vi "Warning Edit.vi"(10 "Data Path":path, 11 "Project":string) -> (2 "Warning Data":string[][](array[string]), 3 "OK?":bool)   [LabVIEW 2020]
uses:
  <vilib>/Utility/miscctls.llb/LVMapReplaceAction.ctl
  <vilib>/Utility/file.llb/Write Delimited Spreadsheet (string).vi
  <vilib>/Utility/file.llb/Read Delimited Spreadsheet (string).vi
panel:
  in  "Warning Group Delete":bool
  in  "Warning Group Add":bool
  in  "WarningGroup":i32(listbox)
  in  "Warning Delete":bool
  in  "Warning Export":bool
  in  "Warning Import":bool
  in  "Warning Edit":bool
  in  "Digital":dbl format="%#.6f"
  in  "level":u16(ring) items=["〇", "Ⅰ", "Ⅱ", "Ⅲ"]
  in  "Warning List":i32(listbox) caption="报警日志"
  in  "OK":bool
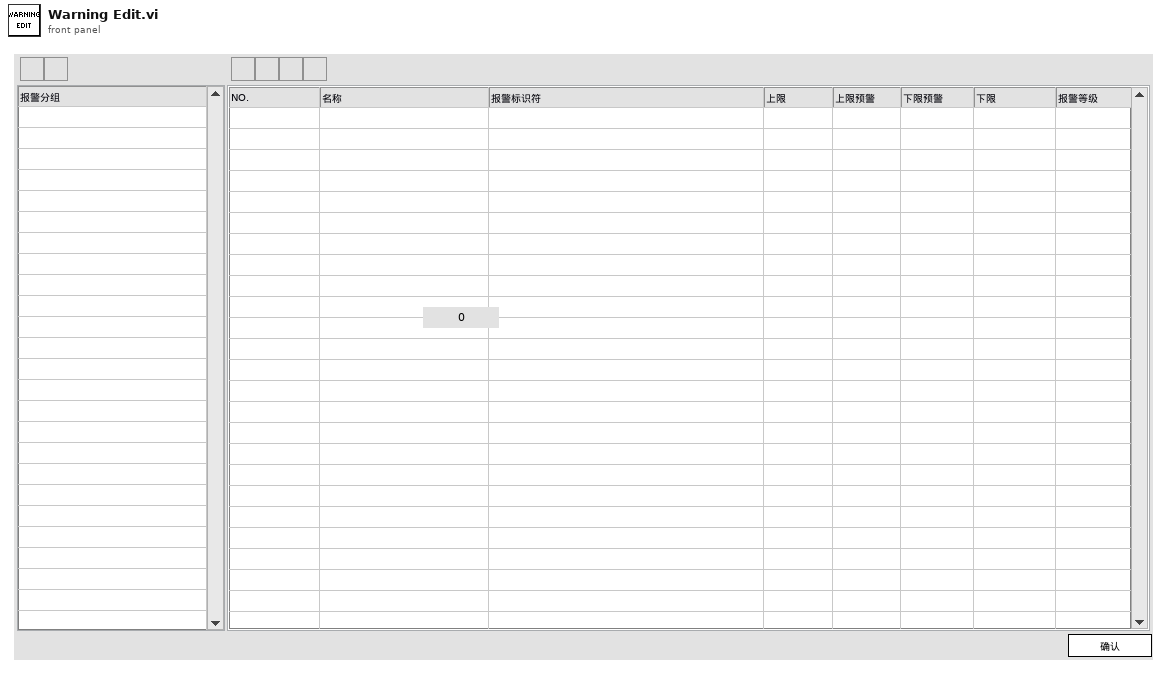
[diagram p1: front panel]
types:
  T1 = typedef "LVPoint32TypeDef.ctl" = cluster{"Horizontal":i32, "Vertical":i32}
  T2 = typedef "LVRowAndColumnTypeDef.ctl" = cluster{"Row":i32, "Column":i32}
  T3 = typedef "LVPositionTypeDef.ctl" = cluster{"Left":i32, "Top":i32}
  T4 = cluster{"Project":string, "Warning List":string[][], "OK?":bool, "Warning":map{string, cluster{"Name":string, "ID":string, "UpperLimit":dbl, "UpperWarning":dbl, "LowerLimit":dbl, "LowerWarning":dbl, "level":enum16{"", "Ⅰ", "Ⅱ", "Ⅲ"}}}, "Data Path":path, "Warning0":refnum<vi>, "WarningContent":refnum<vi>, "Formular List0":string[], "Value":i32}
  T5 = typedef "LVMapReplaceAction.ctl" = enum32{"Modify Entry only if found", "Add or Modify Entry", "Delete Entry"}
  T6 = map{string, cluster{"Name":string, "ID":string, "UpperLimit":dbl, "UpperWarning":dbl, "LowerLimit":dbl, "LowerWarning":dbl, "level":enum16{"", "Ⅰ", "Ⅱ", "Ⅲ"}}}
  T7 = cluster{"Name":string, "ID":string, "UpperLimit":dbl, "UpperWarning":dbl, "LowerLimit":dbl, "LowerWarning":dbl, "level":enum16{"", "Ⅰ", "Ⅱ", "Ⅲ"}}
  T8 = typedef "SDQ Data Type.ctl" = cluster{"CAN Length":string, "CAN Name":string, "CAN ID":string, "CAN Type":string, "Test Item":string, "Byte Order":string, "Instruction":string, "Control Type":string, "Group":string, "Offset":dbl, "Coefficient":dbl, "Write Enable":bool, "Lable Type":string, "Key?":string, "Set Value":string, "Upper":dbl, "Lower":dbl, "Unit":string, "Formula":string, "Test Item Type":string, "Length":i32, "Address":string, "Name":string, "Identifier":string, "Data Type":string, "Enumerate?":string, "Enumerate List":string, "Data":string, "Source":string}
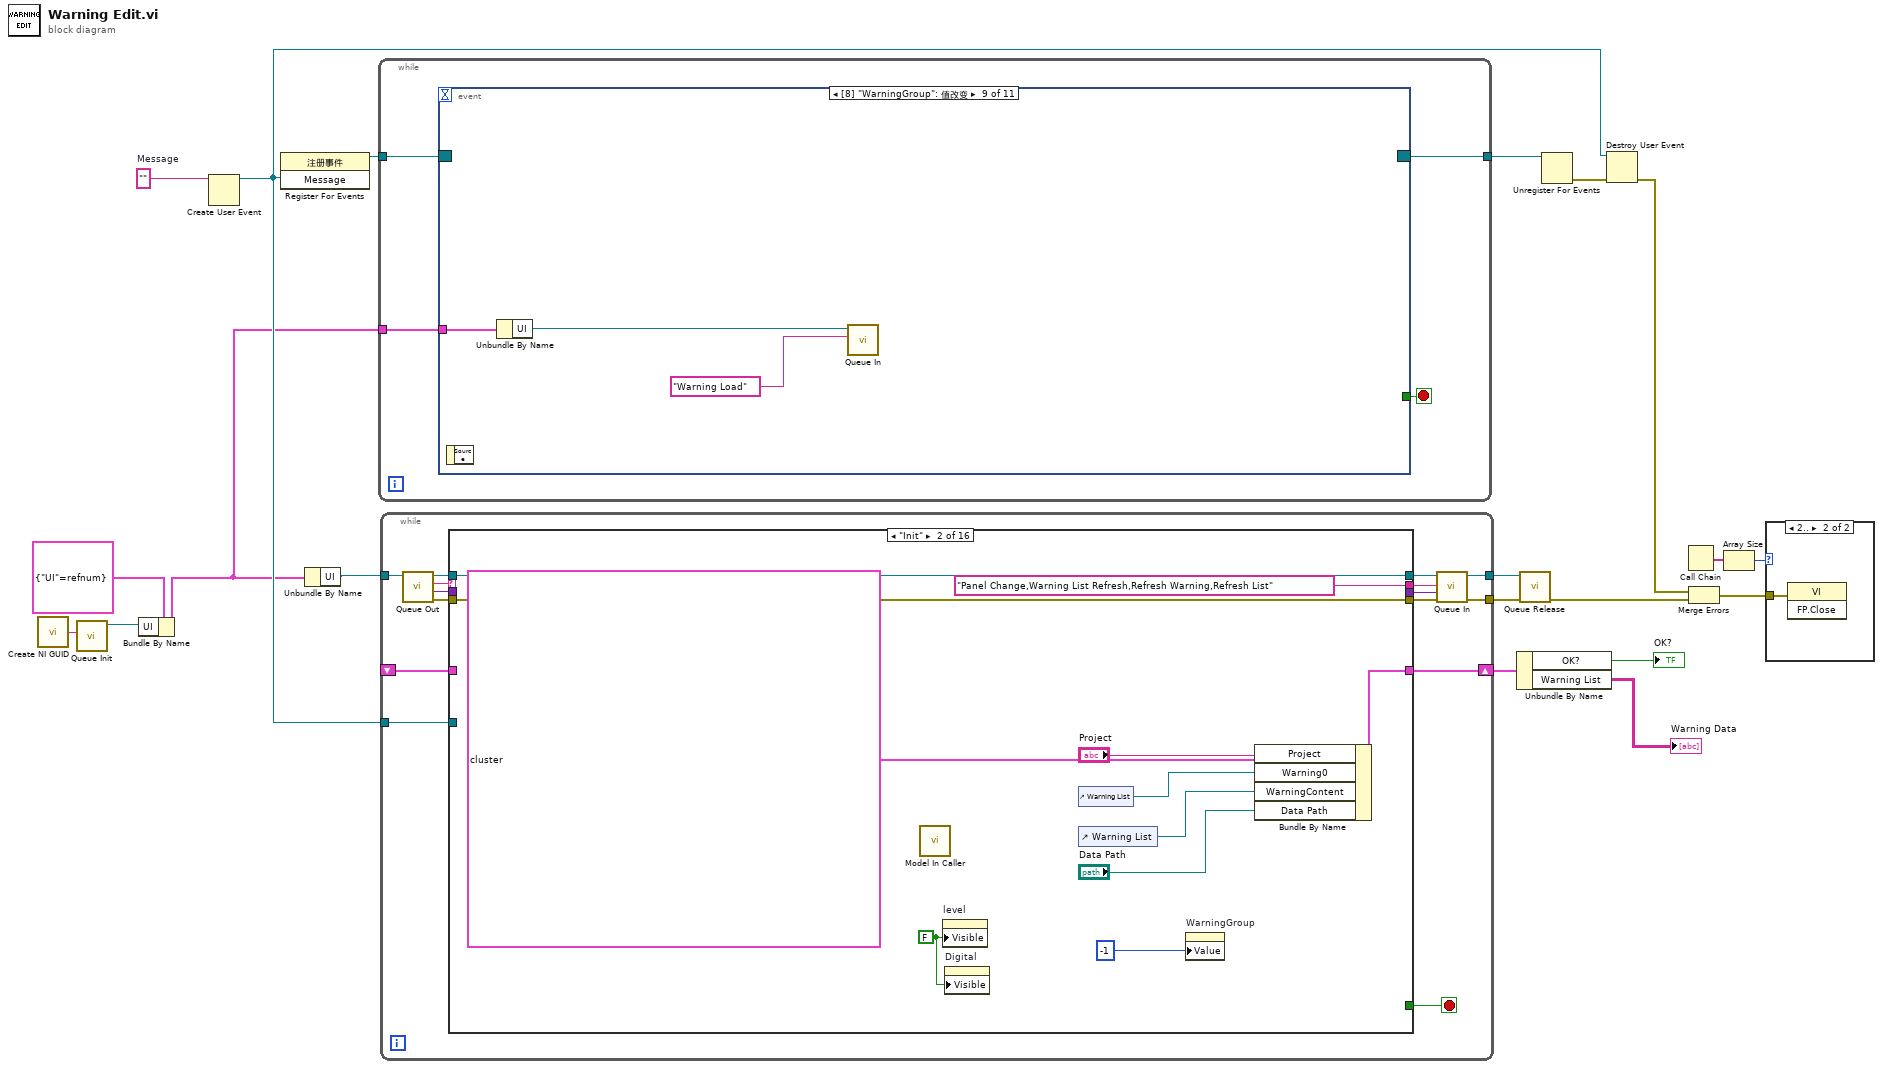
[diagram p0: block diagram]
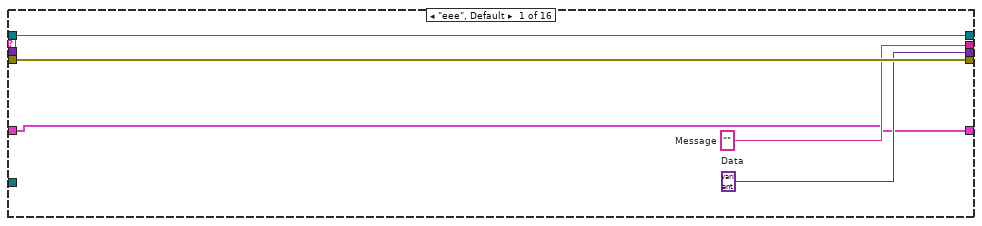
[diagram p3: hidden frame]
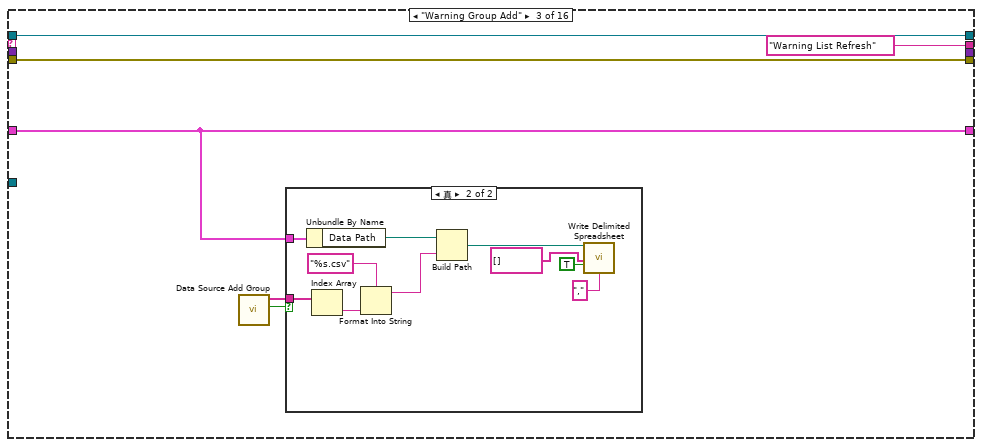
[diagram p4: hidden frame]
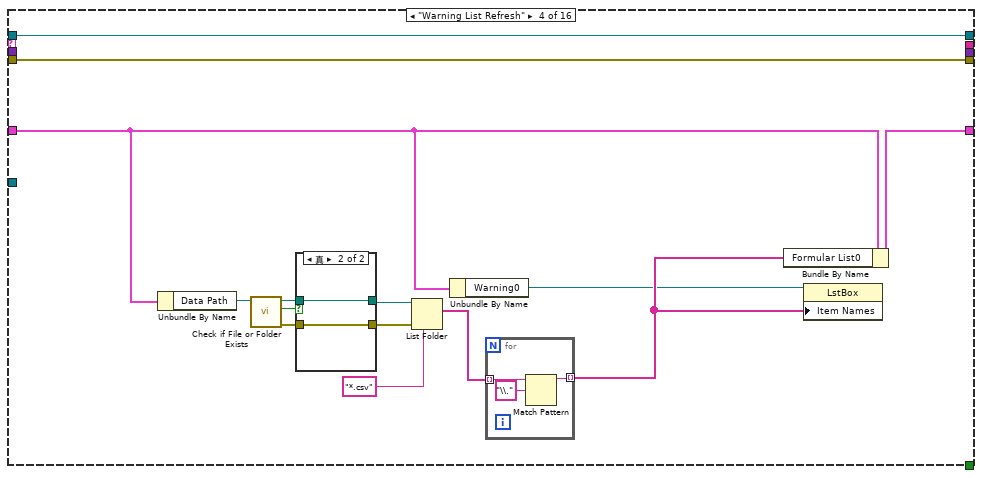
[diagram p6: hidden frame]
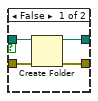
[diagram p7: hidden frame]
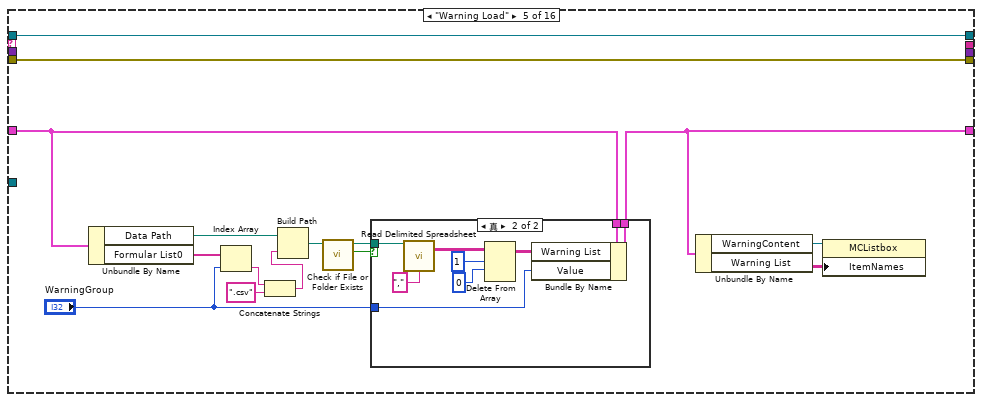
[diagram p8: hidden frame]
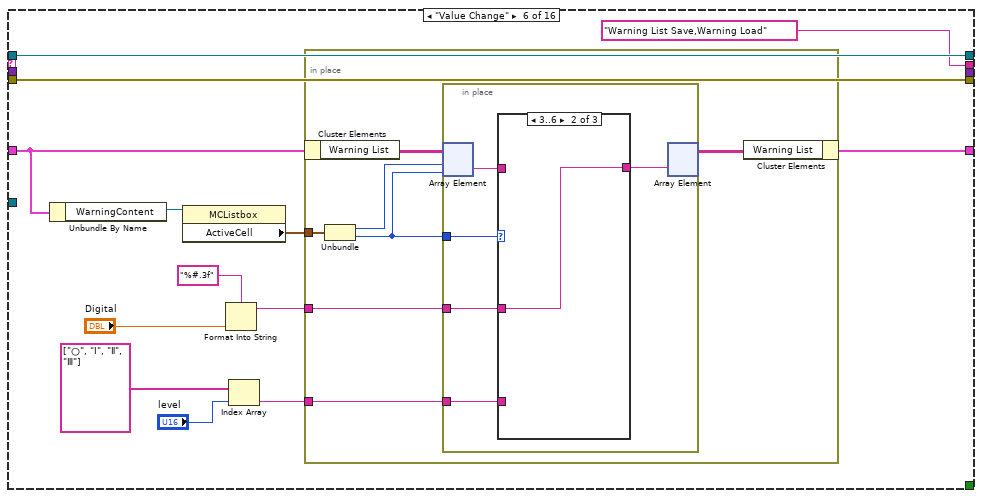
[diagram p10: hidden frame]
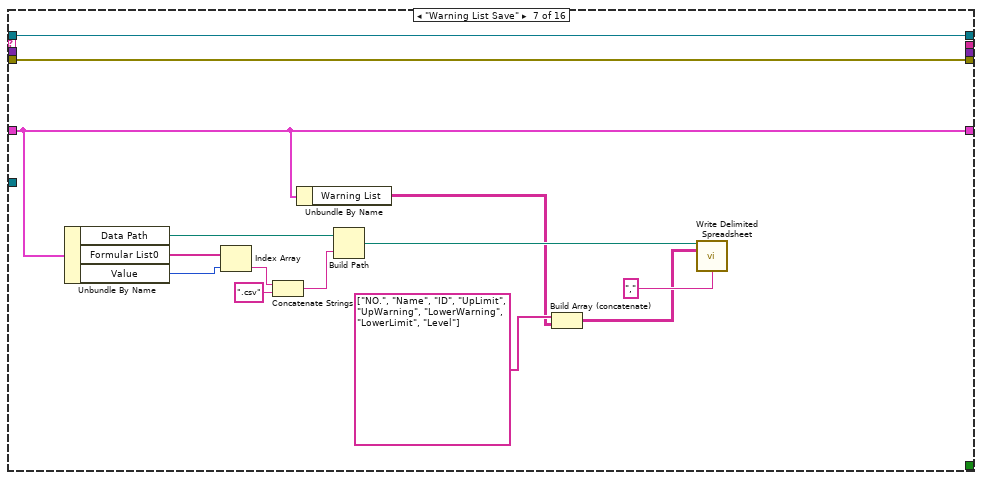
[diagram p13: hidden frame]
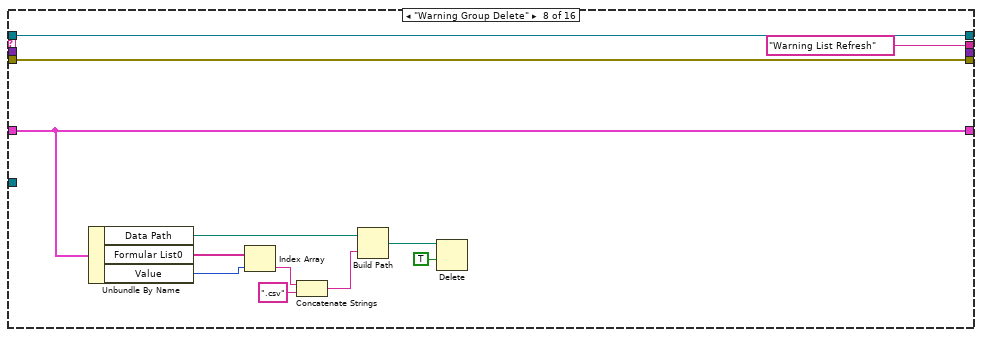
[diagram p14: hidden frame]
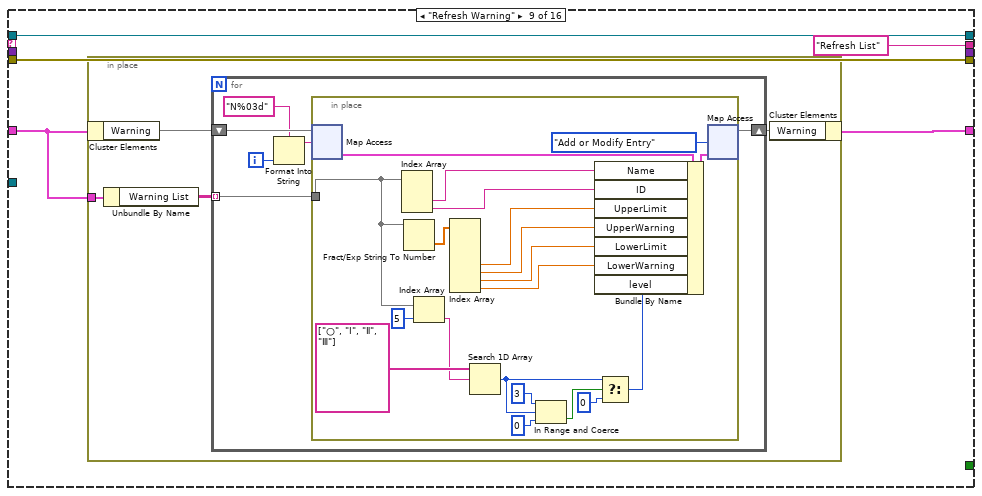
[diagram p15: hidden frame]
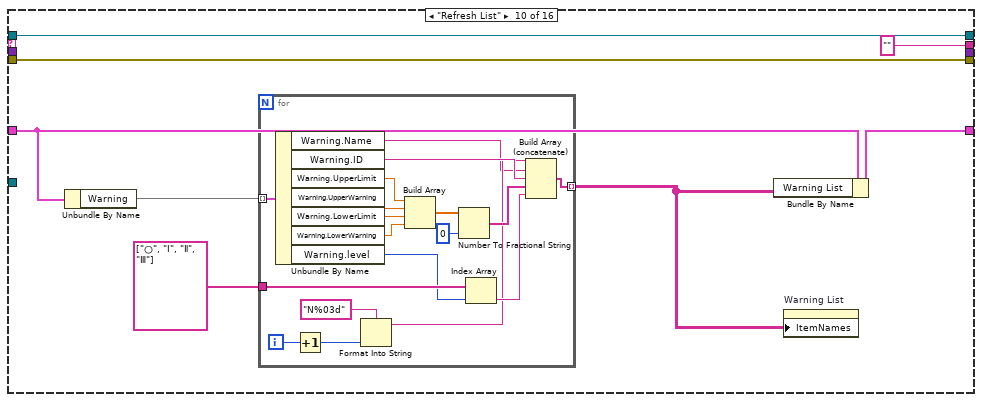
[diagram p16: hidden frame]
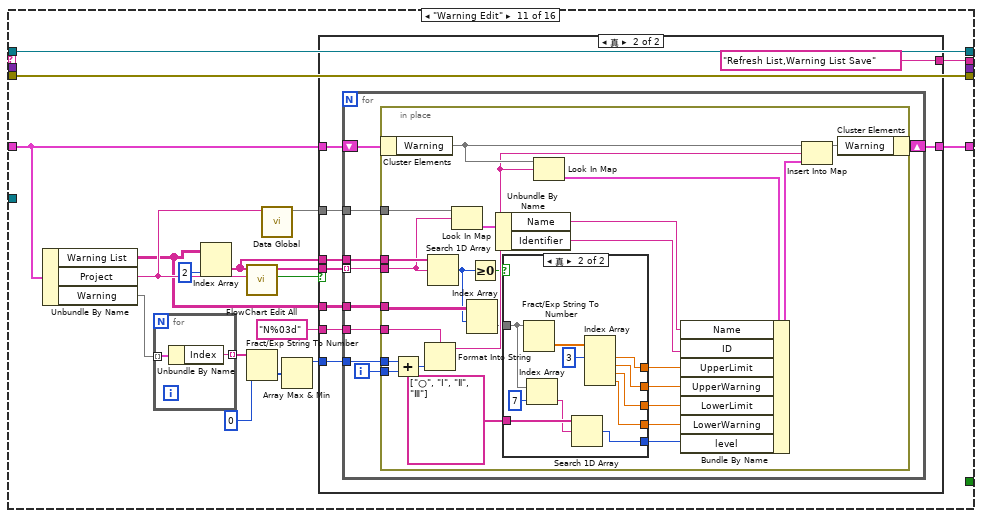
[diagram p17: hidden frame]
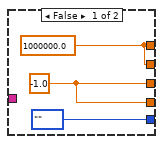
[diagram p19: hidden frame]
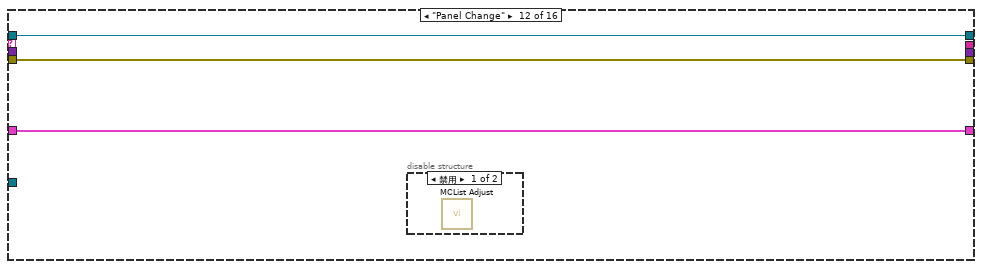
[diagram p20: hidden frame]
diagram:
  w8 = ""  # Message
  n1 = call <vilib>:"Create NI GUID.vi"() -> ("NI GUID"=w6:string)
  n2 = call "Queue Init.vi"("Queue Name"=w6) -> ("Queue Out"=w4:refnum<queue>)  [unwired: 8 in, 2 out]
  n3 = Bundle By Name(cluster=cluster{"UI":refnum<queue>} {"UI"=refnum} ("Queue Ref Out"), "UI"=w4) -> (w5:cluster{"UI":refnum<queue>})
  n4 = Create User Event(user event datatype=w8) -> (user event=w12:refnum<user-event>)  [unwired: 1 in, 1 out]
  n5 = register-events(w12) -> (reference out=w9:refnum<event-registration>)  [unwired: 2 in, 1 out]
  n6 = Unbundle By Name(w5) -> ("UI"=w15:refnum<queue>)
  n7 = while {
    tunnel: w9 -> [w24]
    tunnel: [w22] -> w10
    tunnel: w5 -> [w21]
    stop <- w23 stop-if-true
    n8 = event shown="[8] \"WarningGroup\": 值改变" {
      selector: w24 -> [_ _ _ _ _ _ _ _ _ _ _]
      dyn-events: [_ _ _ _ _ _ _ _ _ _ _] -> w22
      timeout: _ -> [_ _ _ _ _ _ _ _ _ _ _]
      tunnel: [_ _ _ _ w36 _ _ _ _ _ _] -> w23
      tunnel: w21 -> [_ _ w31 w34 _ w41 w46 w49 w52 _ w94]
      event Timeout {
        n9 = event-data() -> ()  [unwired: 1 in, 1 out]
      }
      event Key Down {
        n10 = event-data() -> ("Char"=w26:i16, "PlatMods.Ctrl"=w25:bool)  [unwired: 1 in]
        n11 = case shown="真" w25 {
          tunnel: w26 -> [_ w27]
          frame False {
          }
          frame True {
            n12 = case shown="101" w27 {
              frame 0, Default {
              }
              frame 101 {
                n13 = property class="VI"("BDWin.Open"=TRUE ("程序框图窗口:打开")) -> ()  [unwired: 2 in, 2 out]
              }
            }
          }
        }
      }
      event Panel Resize {
        n14 = event-data() -> ()  [unwired: 1 in, 1 out]
        n15 = Unbundle By Name(w31) -> ("UI"=w30:refnum<queue>)
        n16 = call "Queue In.vi"("Message"="Panel Change", "Queue In"=w30) -> ()  [unwired: 8 in, 2 out]
      }
      event "OK": Value Change {
        n17 = event-data() -> ("CtlRef"=w35:refnum<vi>)  [unwired: 1 in]
        n18 = property class="Bool"(reference=w35) -> ("Label.Text"=w32:string)  [unwired: 1 in, 2 out]
        n19 = Unbundle By Name(w34) -> ("UI"=w33:refnum<queue>)
        n20 = call "Queue In.vi"("Message"=w32, "Queue In"=w33) -> ()  [unwired: 8 in, 2 out]
      }
      event User Event {
        n21 = event-data() -> ("Message"=w38:string)  [unwired: 1 in]
        n22 = Equal?(x=w38, y="Exit") -> (x = y?=w36:bool)
      }
      event Panel Close? {
        n23 = event-data() -> ()  [unwired: 1 in, 1 out]
        n24 = Unbundle By Name(w41) -> ("UI"=w40:refnum<queue>)
        n25 = call "Queue In.vi"("Message"="Exit", "Queue In"=w40) -> ()  [unwired: 8 in, 2 out]
        n26 = event-data("Discard?"=TRUE ("放弃？")) -> ()  [unwired: 1 in, 1 out]
      }
      event "Warning Edit", "Warning Import", "Warning Export", "Warning Delete", "Warning Group Add", "Warning Group Delete": Value Change {
        n27 = event-data() -> ("CtlRef"=w45:refnum<vi>)  [unwired: 1 in]
        n28 = Unbundle By Name(w46) -> ("UI"=w44:refnum<queue>)
        n29 = property class="Bool"(reference=w45) -> ("Label.Text"=w43:string)  [unwired: 1 in, 2 out]
        n30 = call "Queue In.vi"("Message"=w43, "Queue In"=w44) -> ()  [unwired: 8 in, 2 out]
      }
      event "Warning List": Double Click {
        n31 = event-data() -> ()  [unwired: 1 in, 1 out]
        n32 = Unbundle By Name(w49) -> ("UI"=w48:refnum<queue>)
        n33 = call "Queue In.vi"("Message"="Warning Edit", "Queue In"=w48) -> ()  [unwired: 8 in, 2 out]
      }
      event "WarningGroup": Value Change {
        n34 = event-data() -> ()  [unwired: 1 in, 1 out]
        n35 = Unbundle By Name(w52) -> ("UI"=w51:refnum<queue>)
        n36 = call "Queue In.vi"("Message"="Warning Load", "Queue In"=w51) -> ()  [unwired: 8 in, 2 out]
      }
      event "Warning List": Mouse Down {
        n37 = event-data() -> ("CtlRef"=w74:refnum<vi>, "Coords"=w73:T1)  [unwired: 1 in]
        n38 = invoke class="MCListbox (严格)" method="Point To Row Column"(reference=w74, "Point"=w73) -> (reference out=w72:refnum<vi>, "CellPosition"=w68:T2)  [unwired: 5 in, 5 out]
        n39 = property class="MCListbox (严格)"(reference=w72, "ActiveCell"=w68) -> ("ItemNames"=w60:string[][], "Height"=w67:u32, "Width"=w66:u32, "ActiveCellPos"=w65:T3)  [unwired: 1 in, 2 out]
        n40 = Matrix Size(0:w60) -> (1:w71:i32, 2:w69:i32)
        n41 = Unbundle(w68) -> ("Row"=w59:i32, "Column"=w58:i32)
        n42 = Decrement(x=w71) -> (x-1=w64:i32)
        n43 = Greater Or Equal?(x=w64, y=w59) -> (x >= y?=w70:bool)
        n44 = Decrement(x=w69) -> (x-1=w63:i32)
        n45 = Index Array(array=w60, index (row)=w59, index (col)=w58) -> (element=w55:string)
        n46 = case shown="0.." w59 {
          tunnel: w58 -> [_ w79]
          tunnel: w70 -> [_ w78]
          tunnel: w63 -> [_ w77]
          tunnel: [_ w76] -> w61
          tunnel: [_ w75] -> w62
          frame -1, Default {
          }
          frame 0.. {
            n47 = case shown="真" w78 {
              tunnel: w79 -> [_ w83]
              tunnel: w77 -> [_ w84]
              tunnel: [_ w81] -> w76
              tunnel: [_ w80] -> w75
              frame False {
              }
              frame True {
                n48 = Greater Or Equal?(x=w84, y=w83) -> (x >= y?=w82:bool)
                n49 = case shown="真" w82 {
                  tunnel: w83 -> [_ w87]
                  tunnel: [_ w86] -> w81
                  tunnel: [_ w85] -> w80
                  frame False {
                  }
                  frame True {
                    n50 = case shown="7" w87 {
                      tunnel: [_ _ TRUE] -> w86
                      tunnel: [_ TRUE _] -> w85
                      frame 0, Default {
                      }
                      frame 3..6 {
                      }
                      frame 7 {
                      }
                    }
                  }
                }
              }
            }
          }
        }
        n51 = Fract/Exp String To Number(string=w55) -> (number=w57:dbl)  [unwired: 3 in, 1 out]
        n52 = Search 1D Array(1D array=string[] ["〇", "Ⅰ", "Ⅱ", "Ⅲ"], element=w55) -> (index of element=w54:i32)  [unwired: 1 in]
        n53 = expression code="x-5"(w66) -> (w53:u32)
        n54 = property on="Digital" class="DigNum (严格)"("Visible"=w62, "NumText.Height"=w67, "NumText.Width"=w53, "Position"=w65, "Key Focus"=w62, "Value"=w57) -> ()  [unwired: 2 in, 2 out]
        n55 = property on="level" class="Ring (严格)"("Visible"=w61, "Height"=w67, "Width"=w53, "Position"=w65, "Key Focus"=w61, "Value"=w54) -> ()  [unwired: 2 in, 2 out]
      }
      event "Digital", "level": Value Change {
        n56 = event-data() -> ("CtlRef"=w91:refnum<vi>)  [unwired: 1 in]
        n57 = Unbundle By Name(w94) -> ("UI"=w93:refnum<queue>)
        n58 = property class="Num"(reference=w91, "Visible"=FALSE ("可见")) -> ()  [unwired: 1 in, 2 out]
        n59 = call "Queue In.vi"("Message"="Value Change", "Queue In"=w93) -> ()  [unwired: 8 in, 2 out]
      }
    }
  }
  n60 = while {
    tunnel: w15 -> [w104]
    tunnel: [w101] -> w13
    tunnel: [w100] -> w14
    tunnel: w12 -> [w108]
    shift-right: [w96] -> w3
    shift-left: _ -> [w95]
    stop <- w109 stop-if-true
    n61 = call "Queue Out.vi"("Queue In"=w104) -> ("error out"=w107:errorcluster, "Data"=w105:variant, "Message"=w106:string, "Queue Out"=w103:refnum<queue>)  [unwired: 6 in, 1 out]
    n62 = case shown="\"Init\"" w106 {
      selector: w106 -> [_ _ _ _ _ _ _ _ _ _ _ _ _ _ w410 _]
      tunnel: w103 -> [w114 w125 w131 w155 w179 w202 w231 w243 w248 w286 w322 w385 w396 w408 w414 w419]
      tunnel: w107 -> [w113 w124 w130 w154 w178 w201 w230 w242 w247 w285 w321 w384 w395 w407 w412 w420]
      tunnel: [w114 w125 w131 w155 w179 w202 w231 w243 w248 w286 w322 w385 w396 w408 w413 w419] -> w102
      tunnel: [w113 w124 w130 w154 w178 w201 w230 w242 w247 w285 w321 w384 w395 w407 w411 w420] -> w99
      tunnel: [w112 "Panel Change,Warning List Refresh,Refresh Warning,Refresh List" ("Message") "Warning List Refresh" ("Message") _ _ "Warning List Save,Warning Load" ("Message") _ "Warning List Refresh" ("Message") "Refresh List" ("Message") "" ("Message") w310 _ "Exit" ("Message") "Exit" ("Message") "Quit" _] -> w98
      tunnel: [_ _ _ _ _ _ _ _ _ _ _ _ _ _ _ TRUE] -> w109
      tunnel: w108 -> [_ _ _ _ _ _ _ _ _ _ _ _ _ _ w416 _]
      tunnel: [w111 _ _ _ _ _ _ _ _ _ _ _ _ _ _ _] -> w97
      tunnel: w105 -> [_ _ _ _ _ _ _ _ _ _ _ _ _ _ _ _]
      tunnel: [w110 w121 w127 w142 w165 w200 w224 w236 w246 w281 w316 w383 w393 w405 w409 w417] -> w96
      tunnel: w95 -> [w110 _ w127 w143 w167 w198 w224 w236 w245 w284 w317 w383 w391 w405 w409 w417]
      frame "eee", Default {
        w111 = variant  # Data
        w112 = ""  # Message
      }
      frame "Init" {
        w115 = FALSE ("可见")
        n63 = call "Model In Caller.vi"() -> ()  [unwired: 11 in, 1 out]
        n64 = property on="level" class="Ring (严格)"("Visible"=w115) -> ()  [unwired: 2 in, 2 out]
        n65 = property on="Digital" class="DigNum (严格)"("Visible"=w115) -> ()  [unwired: 2 in, 2 out]
        n66 = control-ref of="Warning List"() -> (w119:refnum<vi>)
        n67 = control-ref of="Warning List"() -> (w118:refnum<vi>)
        n68 = property on="WarningGroup" class="LstBox (严格)"("Value"=-1 ("WarningGroup")) -> ()  [unwired: 2 in, 2 out]
        n69 = Bundle By Name(cluster=T4 {"Project"="", "Warning List"=[], "OK?"=FALSE, "Warning"={}, "Data Path"=path "", "Warning0"=refnum, "WarningContent"=refnum, "Formular List0"=[], "Value"=0}, "Project"="Project", "Warning0"=w119, "WarningContent"=w118, "Data Path"="Data Path") -> (w121:T4)
      }
      frame "Warning Group Add" {
        n70 = call "Data Source Add Group.vi"() -> ("OK？"=w129:bool, "Data Out"=w128:string[])  [unwired: 9 in, 1 out]
        n71 = case shown="真" w129 {
          tunnel: w128 -> [_ w141]
          tunnel: w127 -> [_ w140]
          frame False {
          }
          frame True {
            n72 = Unbundle By Name(w140) -> ("Data Path"=w139:path)
            n73 = Index Array(array=w141) -> (element=w137:string)  [unwired: 1 in]
            n74 = Format Into String(format string="%s.csv" ("格式字符串"), w137) -> (resulting string=w136:string)  [unwired: 2 in, 1 out]
            n75 = Build Path(base path=w139, name or relative path=w136) -> (appended path=w135:path)
            n76 = call-poly <vilib>:"Write Delimited Spreadsheet.vi"("file path (dialog if empty)"=w135, "1D data"=string[] [], "append to file? (new file:F)"=TRUE, "delimiter (\\t)"="," ("delimiter (\\t)")) -> ()  [unwired: 10 in, 2 out]
          }
        }
      }
      frame "Warning List Refresh" {
        n77 = Unbundle By Name(w143) -> ("Data Path"=w144:path)
        n78 = call <vilib>:"Check if File or Folder Exists.vi"("path"=w144) -> ("error out"=w147:errorcluster, "file or folder exists?"=w145:bool, "dup path"=w146:path)  [unwired: 8 in]
        n79 = case shown="真" w145 {
          tunnel: w146 -> [w162 w164]
          tunnel: w147 -> [w161 w163]
          tunnel: [w159 w164] -> w148
          tunnel: [w160 w163] -> w149
          frame False {
            n80 = Create Folder(path (use dialog)=w162, error in=w161) -> (created path=w159:path, error out=w160:errorcluster)  [unwired: 1 in, 1 out]
          }
          frame True {
          }
        }
        n81 = List Folder(path=w148, pattern="*.csv" ("类型"), error in=w149) -> (filenames=w152:string[])  [unwired: 1 in, 3 out]
        n82 = Unbundle By Name(w143) -> ("Warning0"=w150:refnum<vi>)
        n83 = for {
          tunnel: w152 -> [w158] mode=indexing
          tunnel: [w156] -> w153 mode=indexing
          n84 = Match Pattern(string=w158, regular expression="\\." ("正则表达式")) -> (before substring=w156:string)  [unwired: 1 in, 3 out]
        }
        n85 = Bundle By Name(cluster=w143, "Formular List0"=w153) -> (w142:T4)
        n86 = property class="LstBox"(reference=w150, "Item Names"=w153) -> ()  [unwired: 1 in, 2 out]
      }
      frame "Warning Load" {
        n87 = Unbundle By Name(w167) -> ("Data Path"=w168:path, "Formular List0"=w174:string[])
        n88 = Index Array(array=w174, index="WarningGroup") -> (element=w175:string)
        n89 = Concatenate Strings(w175, ".csv" ("字符串")) -> (w177:string)
        n90 = Build Path(base path=w168, name or relative path=w177) -> (appended path=w171:path)
        n91 = call <vilib>:"Check if File or Folder Exists.vi"("path"=w171) -> ("file or folder exists?"=w172:bool, "dup path"=w173:path)  [unwired: 8 in, 1 out]
        n92 = case shown="真" w172 {
          tunnel: w167 -> [w180 w189]
          tunnel: [w180 w183] -> w165
          tunnel: "WarningGroup" -> [_ w182]
          tunnel: w173 -> [_ w181]
          frame False {
          }
          frame True {
            n93 = call-poly <vilib>:"Read Delimited Spreadsheet.vi"("file path (dialog if empty)"=w181, "delimiter (\\t)"="," ("delimiter (\\t)")) -> ("all rows"=w184:string[][])  [unwired: 8 in, 5 out]
            n94 = Delete From Array(array=w184, length=1 ("长度"), index (row)=0 ("索引 (行)")) -> (array with subset deleted=w187:string[][])  [unwired: 1 in, 1 out]
            n95 = Bundle By Name(cluster=w189, "Warning List"=w187, "Value"=w182) -> (w183:T4)
          }
        }
        n96 = Unbundle By Name(w165) -> ("WarningContent"=w170:refnum<vi>, "Warning List"=w169:string[][])
        n97 = property on="属性节点" class="MCListbox"(reference=w170, "ItemNames"=w169) -> ()  [unwired: 1 in, 2 out]
      }
      frame "Value Change" {
        n98 = Unbundle By Name(w198) -> ("WarningContent"=w197:refnum<vi>)
        n99 = property class="MCListbox"(reference=w197) -> ("ActiveCell"=w196:T2)  [unwired: 1 in, 2 out]
        n100 = Format Into String(format string="%#.3f" ("格式字符串"), "Digital") -> (resulting string=w193:string)  [unwired: 2 in, 1 out]
        n101 = Index Array(array=string[] ["〇", "Ⅰ", "Ⅱ", "Ⅲ"], index="level") -> (element=w190:string)
        n102 = in-place {
          in-place-border: w196 -> [w208]
          in-place-border: w193 -> [w204]
          in-place-border: w190 -> [w203]
          n103 = in-place-cluster #1(w198) -> ("Warning List"=w209:string[][])
          n104 = Unbundle(w208) -> ("Row"=w207:i32, "Column"=w205:i32)
          n105 = in-place {
            in-place-border: w205 -> [w214]
            in-place-border: w204 -> [w211]
            in-place-border: w203 -> [w210]
            n106 = in-place-array #2(w209, w207, w205) -> (w213:string)
            n107 = case shown="3..6" w214 {
              tunnel: [w215 w216 w217] -> w212
              tunnel: w213 -> [w215 _ _]
              tunnel: w211 -> [_ w216 _]
              tunnel: w210 -> [_ _ w217]
              frame 0, Default {
              }
              frame 3..6 {
              }
              frame 7 {
              }
            }
            n108 = in-place-array #2(w212) -> (w206:string[][])  [unwired: 2 out]
          }
          n109 = in-place-cluster #1("Warning List"=w206) -> (w200:T4)
        }
      }
      frame "Warning List Save" {
        n110 = Unbundle By Name(w224) -> ("Data Path"=w225:path, "Formular List0"=w226:string[], "Value"=w223:i32)
        n111 = Index Array(array=w226, index=w223) -> (element=w227:string)
        n112 = Concatenate Strings(w227, ".csv" ("字符串")) -> (w229:string)
        n113 = Unbundle By Name(w224) -> ("Warning List"=w219:string[][])
        n114 = Build Path(base path=w225, name or relative path=w229) -> (appended path=w221:path)
        n115 = Build Array (concatenate)(string[] ["NO.", "Name", "ID", "UpLimit", "UpWarning", "LowerWarning", "LowerLimit", "Level"], w219) -> (w218:string[][])
        n116 = call-poly <vilib>:"Write Delimited Spreadsheet.vi"("file path (dialog if empty)"=w221, "2D data"=w218, "delimiter (\\t)"="," ("delimiter (\\t)")) -> ()  [unwired: 11 in, 2 out]
      }
      frame "Warning Group Delete" {
        n117 = Unbundle By Name(w236) -> ("Data Path"=w237:path, "Formular List0"=w238:string[], "Value"=w235:i32)
        n118 = Index Array(array=w238, index=w235) -> (element=w239:string)
        n119 = Concatenate Strings(w239, ".csv" ("字符串")) -> (w241:string)
        n120 = Build Path(base path=w237, name or relative path=w241) -> (appended path=w234:path)
        n121 = Delete(path (use dialog)=w234, confirm (F)=TRUE ("确认(F)")) -> ()  [unwired: 3 in, 3 out]
      }
      frame "Refresh Warning" {
        n122 = in-place {
          in-place-border: w245 -> [w252]
          n123 = in-place-cluster #3(w245) -> ("Warning"=w250:T6)
          n124 = Unbundle By Name(w252) -> ("Warning List"=w251:string[][])
          n125 = for {
            tunnel: w251 -> [w253] mode=indexing
            shift-right: [w257] -> w249
            shift-left: w250 -> [w258]
            i -> [w255]
            n126 = Format Into String(format string="N%03d" ("格式字符串"), w255) -> (resulting string=w254:string)  [unwired: 2 in, 1 out]
            n127 = in-place {
              in-place-border: w253 -> [w270]
              n128 = in-place-map #4(w258, w254) -> (w278:T7)  [unwired: 1 in, 1 out]
              n129 = Index Array(array=w270) -> (element #2=w260:string, element #3=w259:string)  [unwired: 3 in, 1 out]
              n130 = Fract/Exp String To Number(string=w270) -> (number=w275:dbl[])  [unwired: 3 in, 1 out]
              n131 = Index Array(array=w270, index=5 ("索引")) -> (element=w262:string)
              n132 = Index Array(array=w275) -> (element #4=w274:dbl, element #5=w273:dbl, element #6=w272:dbl, element #7=w271:dbl)  [unwired: 7 in, 3 out]
              n133 = Search 1D Array(1D array=string[] ["〇", "Ⅰ", "Ⅱ", "Ⅲ"], element=w262) -> (index of element=w268:i32)  [unwired: 1 in]
              n134 = In Range and Coerce(upper limit=3 ("上限"), x=w268, lower limit=0 ("下限")) -> (In Range?=w267:bool)  [unwired: 1 out]
              n135 = Select(t=w268, s=w267, f=0) -> (s? t:f=w261:i32)
              n136 = Bundle By Name(cluster=w278, "Name"=w260, "ID"=w259, "UpperLimit"=w274, "UpperWarning"=w273, "LowerLimit"=w272, "LowerWarning"=w271, "level"=w261) -> (w276:T7)
              n137 = in-place-map #4(w276, LVMapReplaceAction."Add or Modify Entry" ("操作")) -> (w257:T6)  [unwired: 2 out]
            }
          }
          n138 = in-place-cluster #3("Warning"=w249) -> (w246:T4)
        }
      }
      frame "Refresh List" {
        n139 = Unbundle By Name(w284) -> ("Warning"=w283:T6)
        n140 = for {
          tunnel: w283 -> [w304] mode=indexing
          tunnel: string[] ["〇", "Ⅰ", "Ⅱ", "Ⅲ"] -> [w295]
          tunnel: [w292] -> w280 mode=indexing
          i -> [w290]
          n141 = Unbundle By Name(w304) -> ("Warning.Name"=w287:string, "Warning.ID"=w297:string, "Warning.UpperLimit"=w303:dbl, "Warning.UpperWarning"=w302:dbl, "Warning.LowerLimit"=w301:dbl, "Warning.LowerWarning"=w300:dbl, "Warning.level"=w294:enum16{"", "Ⅰ", "Ⅱ", "Ⅲ"})
          n142 = Increment(x=w290) -> (x+1=w289:i32)
          n143 = Format Into String(format string="N%03d" ("格式字符串"), w289) -> (resulting string=w288:string)  [unwired: 2 in, 1 out]
          n144 = Build Array(w303, w302, w301, w300) -> (w299:dbl[])
          n145 = Number To Fractional String(number=w299, precision (6)=i16 0 ("精度(6)")) -> (F-format string=w296:string[])  [unwired: 2 in]
          n146 = Index Array(array=w295, index=w294) -> (element=w293:string)
          n147 = Build Array (concatenate)(w288, w287, w297, w296, w293) -> (w292:string[])
        }
        n148 = Bundle By Name(cluster=w284, "Warning List"=w280) -> (w281:T4)
        n149 = property on="Warning List" class="MCListbox (严格)"("ItemNames"=w280) -> ()  [unwired: 2 in, 2 out]
      }
      frame "Warning Edit" {
        n150 = Unbundle By Name(w317) -> ("Warning List"=w306:string[][], "Project"=w309:string, "Warning"=w315:T6)
        n151 = for {
          tunnel: w315 -> [w324] mode=indexing
          tunnel: [w323] -> w314 mode=indexing
          n152 = Unbundle By Name(w324) -> ("Index"=w323:string)
        }
        n153 = Index Array(array=w306, index (col)=2 ("禁用的索引 (列)")) -> (element=w307:string[])  [unwired: 1 in]
        n154 = call "FlowChart Edit All.vi"("Name"=w309, "Identifier In"=w307) -> ("OK？"=w320:bool, "Identifiers Out"=w319:string[])  [unwired: 8 in]
        n155 = Fract/Exp String To Number(string=w314, default (0 dbl)=0 ("默认(0 DBL)")) -> (number=w313:i32[])  [unwired: 2 in, 1 out]
        n156 = call "Data Global.vi"("Name"=w309) -> ("Data Out"=w308:map{string, T8})  [unwired: 7 in, 3 out]
        n157 = Array Max & Min(array=w313) -> (max value=w312:i32)  [unwired: 3 out]
        n158 = case shown="真" w320 {
          tunnel: w319 -> [_ w332]
          tunnel: w317 -> [w325 w334]
          tunnel: [w325 w333] -> w316
          tunnel: w312 -> [_ w331]
          tunnel: [_ "Refresh List,Warning List Save"] -> w310
          tunnel: w308 -> [_ w329]
          tunnel: w307 -> [_ w328]
          tunnel: w306 -> [_ w327]
          tunnel: "N%03d" ("格式字符串") -> [_ w326]
          frame False {
          }
          frame True {
            n159 = for {
              tunnel: w332 -> [w341] mode=indexing
              tunnel: w331 -> [w340]
              shift-right: [w342] -> w333
              shift-left: w334 -> [w343]
              tunnel: w329 -> [w338]
              tunnel: w328 -> [w337]
              tunnel: w327 -> [w336]
              tunnel: w326 -> [w335]
              i -> [w339]
              n160 = in-place {
                in-place-border: w341 -> [w352]
                in-place-border: w340 -> [w364]
                in-place-border: w339 -> [w362]
                in-place-border: w338 -> [w357]
                in-place-border: w337 -> [w353]
                in-place-border: w336 -> [w350]
                in-place-border: w335 -> [w349]
                n161 = in-place-cluster #5(w343) -> ("Warning"=w368:T6)
                n162 = Add(x=w364, y=w362) -> (x+y=w363:i32)
                n163 = Format Into String(format string=w349, w363) -> (resulting string=w358:string)  [unwired: 2 in, 1 out]
                n164 = Search 1D Array(1D array=w353, element=w352) -> (index of element=w348:i32)  [unwired: 1 in]
                n165 = Look In Map(map=w357, key=w352) -> (value=w356:T8)  [unwired: 1 in, 1 out]
                n166 = Index Array(array=w350, index (row)=w348) -> (element=w347:string[])  [unwired: 1 in]
                n167 = Greater Or Equal To 0?(x=w348) -> (x >= 0?=w351:bool)
                n168 = Unbundle By Name(w356) -> ("Name"=w355:string, "Identifier"=w354:string)
                n169 = case shown="真" w351 {
                  tunnel: [w370 w381] -> w361
                  tunnel: [w369 w379] -> w360
                  tunnel: [enum16{"", "Ⅰ", "Ⅱ", "Ⅲ"}."" ("level") w374] -> w359
                  tunnel: w347 -> [_ w376]
                  tunnel: [w370 w380] -> w346
                  tunnel: [w369 w378] -> w345
                  tunnel: string[] ["〇", "Ⅰ", "Ⅱ", "Ⅲ"] -> [_ w377]
                  frame False {
                    w369 = -1.0 ("LowerLimit")
                    w370 = 1000000.0 ("UpperLimit")
                  }
                  frame True {
                    n170 = Fract/Exp String To Number(string=w376) -> (number=w382:dbl[])  [unwired: 3 in, 1 out]
                    n171 = Index Array(array=w376, index=7 ("索引")) -> (element=w375:string)
                    n172 = Search 1D Array(1D array=w377, element=w375) -> (index of element=w374:i32)  [unwired: 1 in]
                    n173 = Index Array(array=w382, index #1=3 ("索引")) -> (element #1=w381:dbl, element #2=w380:dbl, element #3=w379:dbl, element #4=w378:dbl)  [unwired: 3 in]
                  }
                }
                n174 = Look In Map(map=w368, key=w358) -> (value=w366:T7)  [unwired: 1 in, 1 out]
                n175 = Bundle By Name(cluster=w366, "Name"=w355, "ID"=w354, "UpperLimit"=w361, "UpperWarning"=w346, "LowerLimit"=w360, "LowerWarning"=w345, "level"=w359) -> (w365:T7)
                n176 = Insert Into Map(map in=w368, key=w358, value=w365) -> (map out=w367:T6)  [unwired: 2 out]
                n177 = in-place-cluster #5("Warning"=w367) -> (w342:T4)
              }
            }
          }
        }
      }
      frame "Panel Change" {
        n178 = disable-structure shown="禁用" {
          frame Disabled {
            n179 = call "MCList Adjust.vi"() -> ()  [unwired: 11 in, 1 out]
          }
          frame Enabled {
          }
        }
      }
      frame "OK" {
        n180 = Unbundle By Name(w391) -> ("Data Path"=w390:path)
        n181 = List Folder(path=w390, pattern="*.csv" ("类型")) -> (path out=w388:path, filenames=w389:string[])  [unwired: 2 in, 2 out]
        n182 = for {
          tunnel: w389 -> [w403] mode=indexing
          tunnel: w388 -> [w404]
          tunnel: [w397] -> w387 mode=concatenating
          n183 = Build Path(base path=w404, name or relative path=w403) -> (appended path=w402:path)
          n184 = call-poly <vilib>:"Read Delimited Spreadsheet.vi"("file path (dialog if empty)"=w402, "delimiter (\\t)"="," ("delimiter (\\t)")) -> ("all rows"=w400:string[][])  [unwired: 8 in, 5 out]
          n185 = Delete From Array(array=w400, length=1 ("长度"), index (row)=0 ("索引 (行)")) -> (array with subset deleted=w397:string[][])  [unwired: 1 in, 1 out]
        }
        n186 = Bundle By Name(cluster=w391, "OK?"=TRUE, "Warning List"=w387) -> (w393:T4)
      }
      frame "Cancle" {
      }
      frame "Exit" {
        n187 = Generate User Event(user event=w416, event data cluster=w410) -> ()  [unwired: 2 in, 2 out]
        n188 = call "Queue Clear.vi"("error in (no error)"=w412, "Queue In"=w414) -> ("error out"=w411:errorcluster, "Queue Out"=w413:refnum<queue>)  [unwired: 8 in]
      }
      frame "Quit" {
      }
    }
    n189 = call "Queue In.vi"("error in (no error)"=w99, "Data"=w97, "Message"=w98, "Queue In"=w102) -> ("error out"=w100:errorcluster, "Queue Out"=w101:refnum<queue>)  [unwired: 6 in]
  }
  n190 = Unbundle By Name(w3) -> ("OK?"=→"OK?":bool, "Warning List"=→"Warning Data":string[][])
  n191 = call "Queue Release.vi"("error in (no error)"=w14, "Queue In"=w13) -> ("error out"=w17:errorcluster)  [unwired: 9 in]
  n192 = Unregister For Events(event registration refnum=w10) -> (error out=w11:errorcluster)  [unwired: 1 in]
  n193 = Destroy User Event(user event=w12, error in=w11) -> (error out=w16:errorcluster)
  n194 = Call Chain() -> (call chain=w19:string[])
  n195 = Merge Errors(w16, w17) -> (w18:errorcluster)
  n196 = Array Size(array=w19) -> (size(s)=w20:i32)
  n197 = case shown="2.." w20 {
    tunnel: w18 -> [_ w421]
    frame 0, Default {
    }
    frame 2.. {
      n198 = invoke class="VI" method="FP.Close"(error in=w421) -> ()  [unwired: 2 in, 3 out]
    }
  }
